vi "Set PDO recive mapping.vi"(6 "PDO mapping":u32[](array[numeric]), 7 "timeout (1s)":dbl=1.0 min=0.0, 8 "error in (no error)":errorcluster, 9 "PDO channel":u8(ring) items=["PDO 1", "PDO 2", "PDO 3", "PDO 4"], 11 "SDO object in":refnum<k20>) -> (0 "error out":errorcluster, 1 "completion code":u32, 3 "SDO object out":refnum<k20>)   [LabVIEW 2016]
uses:
  <vilib>/CANopenLib/CANOPEN.llb/CANopen SDO Write [U32].vi
  <vilib>/CANopenLib/CANOPEN.llb/CANopen SDO Write [U8].vi
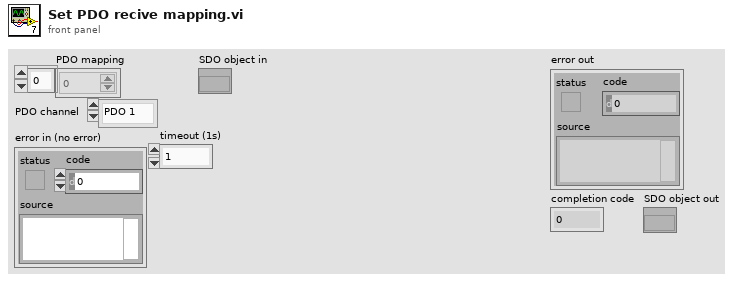
[diagram p1: front panel]
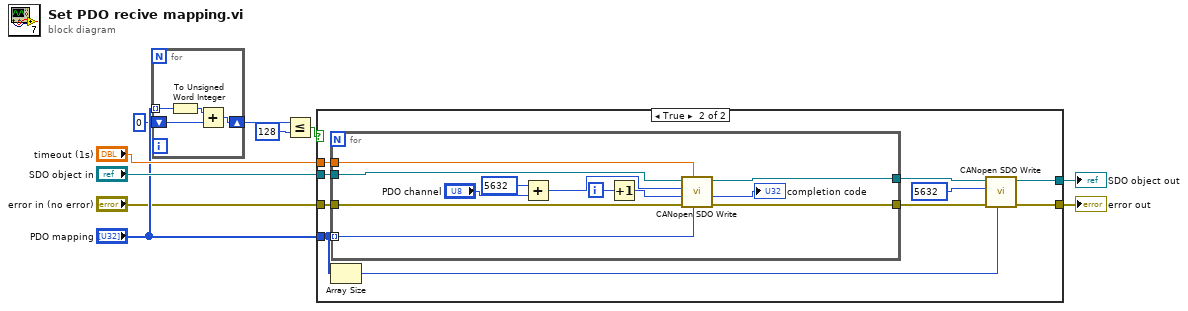
[diagram p0: block diagram]
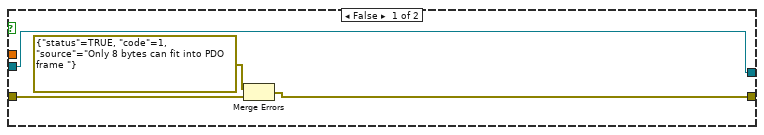
[diagram p2: hidden frame]
diagram:
  n1 = for {
    tunnel: "PDO mapping" -> [w13] mode=indexing
    shift-right: [w12] -> w5
    shift-left: u16 0 -> [w11]
    n2 = To Unsigned Word Integer(number=w13) -> (unsigned 16bit integer=w14:u16)
    n3 = Add(x=w14, y=w11) -> (x+y=w12:u16)
  }
  n4 = Less Or Equal?(x=w5, y=u16 128) -> (x <= y?=w3:bool)
  n5 = case shown="True" w3 {
    tunnel: "PDO mapping" -> [_ w25]
    tunnel: "timeout (1s)" -> [_ w28]
    tunnel: "SDO object in" -> [w16 w27]
    tunnel: [w16 w20] -> w8
    tunnel: [w17 w19] -> w7
    tunnel: "error in (no error)" -> [w15 w26]
    frame False {
      n6 = Merge Errors(errorcluster {"status"=TRUE, "code"=1, "source"="Only 8 bytes can fit into PDO frame "} ("error constant"), w15) -> (w17:errorcluster)
    }
    frame True {
      n7 = for {
        tunnel: w25 -> [w35] mode=indexing
        tunnel: w28 -> [w34]
        tunnel: w27 -> [w33]
        tunnel: [w32] -> w21
        tunnel: [w30] -> w23
        tunnel: w26 -> [w29]
        i -> [w37]
        n8 = Add(x=u16 5632, y="PDO channel") -> (x+y=w38:u16)
        n9 = Increment(x=w37) -> (x+1=w36:i32)
        n10 = call-poly <vilib>:"CANopen SDO Write.vi"("U32 data"=w35, "timeout (1s)"=w34, "error in (no error)"=w29, "object sub-index (0)"=w36, "object index"=w38, "SDO object in"=w33) -> ("error out"=w30:errorcluster, "completion code"=→"completion code":u32, "SDO object out"=w32:refnum<k20>)  [unwired: 3 in]
      }
      n11 = Array Size(array=w25) -> (size(s)=w24:i32)
      n12 = call-poly <vilib>:"CANopen SDO Write.vi"("U8 data"=w24, "error in (no error)"=w23, "object index"=u16 5632, "SDO object in"=w21) -> ("error out"=w19:errorcluster, "SDO object out"=w20:refnum<k20>)  [unwired: 5 in, 1 out]
    }
  }
  "error out" <- w7
  "SDO object out" <- w8
